vi "Dot_Plot_Sub.vi"(8 "Scaler plotted":string, 11 "Data":dbl[][](array[numeric])=[[-106.4208, 283.2907, 10.0, -0.027074, 202.4772, -73.9844, 9.9544], [-106.4108, 183.2989, 10.0, -0.06373, 202.4772, -73.9844, 9.9544], [-106.4104, 233.2978, 10.0, -0.10129, 202.4772, -73.9844, 9.9544], [-106.408, 333.302, 10.0, -0.09306, 202.4772, -73.9844, 9.9544], [138.8906, 606.731, 10.0, -0.003285, 202.4772, -73.9844, 9.9544], [238.889, 47.6577, 10.0, 0.004673, 202.4772, -73.9844, 9.9544], [238.8902, 606.729, 10.0, -0.003458, 202.4772, -73.9844, 9.9544], [288.8878, 47.6581, 10.0, 0.007221, 202.4772, -73.9844, 9.9544], [338.888, 606.73, 10.0, 0.004362, 202.4772, -73.9844, 9.9544], [338.891, 47.6626, 10.0, 0.006298, 202.4772, -73.9844, 9.9544], [388.892, -63.3583, 10.0, 4.5324, 202.4772, -73.9844, 9.9544], [388.892, 47.6606, 10.0, -0.008191, 202.4772, -73.9844, 9.9544], [438.889, 606.729, 10.0, -0.0028755, 202.4772, -73.9844, 9.9544], [438.89, -63.3577, 10.0, 4.2681, 202.4772, -73.9844, 9.9544], [438.891, 47.6608, 10.0, 0.026059, 202.4772, -73.9844, 9.9544], [488.89, 47.6614, 10.0, 0.14972, 202.4772, -73.9844, 9.9544], [488.892, -63.3599, 10.0, 6.2235, 202.4772, -73.9844, 9.9544], [538.89, -63.3596, 10.0, 7.0971, 202.4772, -73.9844, 9.9544], [538.891, 47.6597, 10.0, 0.7831, 202.4772, -73.9844, 9.9544], [538.893, 606.731, 10.0, 0.004097, 202.4772, -73.9844, 9.9544], [588.889, -63.3589, 10.0, 9.8267, 202.4772, -73.9844, 9.9544], [588.89, 47.659, 10.0, 1.4958, 202.4772, -73.9844, 9.9544], [638.889, 47.6597, 10.0, 2.7164, 202.4772, -73.9844, 9.9544], [638.89, 606.731, 10.0, 0.0016489, 202.4772, -73.9844, 9.9544], [638.891, -63.361, 10.0, 9.6904, 202.4772, -73.9844, 9.9544], [688.89, -63.3603, 10.0, 10.7752, 202.4772, -73.9844, 9.9544], [688.89, 47.6576, 10.0, 4.0933, 202.4772, -73.9844, 9.9544], [738.888, -63.3603, 10.0, 9.798, 202.4772, -73.9844, 9.9544], [738.889, 47.6583, 10.0, 5.4641, 202.4772, -73.9844, 9.9544], [738.89, 606.73, 10.0, 0.03667, 202.4772, -73.9844, 9.9544], [788.888, 47.659, 10.0, 6.5562, 202.4772, -73.9844, 9.9544], [788.889, -63.3624, 10.0, 9.7284, 202.4772, -73.9844, 9.9544], [838.888, -63.3617, 10.0, 9.2828, 202.4772, -73.9844, 9.9544], [838.888, 606.731, 10.0, 0.10792, 202.4772, -73.9844, 9.9544], [838.889, 47.6562, 10.0, 6.9452, 202.4772, -73.9844, 9.9544], [888.892, 47.6611, 10.0, 6.813, 202.4772, -73.9844, 9.9544], [888.892, -63.3575, 10.0, 8.8351, 202.4772, -73.9844, 9.9544], [938.888, 606.729, 10.0, 0.5974, 202.4772, -73.9844, 9.9544], [938.891, 47.6618, 10.0, 5.8719, 202.4772, -73.9844, 9.9544], [938.892, -63.3596, 10.0, 8.3492, 202.4772, -73.9844, 9.9544], [988.889, 47.6618, 10.0, 4.8748, 202.4772, -73.9844, 9.9544], [988.891, -63.3589, 10.0, 7.5502, 202.4772, -73.9844, 9.9544], [1038.888, 297.6587, 10.0, 3.1165, 202.4772, -73.9844, 9.9544], [1038.888, 97.6613, 10.0, 4.0692, 202.4772, -73.9844, 9.9544], [1038.888, 222.6594, 10.0, 2.9843, 202.4772, -73.9844, 9.9544], [1038.889, 147.6602, 10.0, 3.7073, 202.4772, -73.9844, 9.9544], [1038.889, 272.6583, 10.0, 3.0147, 202.4772, -73.9844, 9.9544], [1038.89, 72.6609, 10.0, 4.1188, 202.4772, -73.9844, 9.9544], [1038.89, 122.659, 10.0, 3.9763, 202.4772, -73.9844, 9.9544], [1038.89, 197.659, 10.0, 3.099, 202.4772, -73.9844, 9.9544], [1038.89, 247.6571, 10.0, 2.9194, 202.4772, -73.9844, 9.9544], [1038.89, 322.657, 10.0, 2.9534, 202.4772, -73.9844, 9.9544], [1038.89, 572.66, 10.0, 1.2565, 202.4772, -73.9844, 9.9544], [1038.89, 172.6578, 10.0, 3.3414, 202.4772, -73.9844, 9.9544], [1038.89, 447.662, 10.0, 2.4811, 202.4772, -73.9844, 9.9544], [1038.89, 522.662, 10.0, 1.3205, 202.4772, -73.9844, 9.9544], [1038.89, 47.6597, 10.0, 4.5287, 202.4772, -73.9844, 9.9544], [1038.89, -63.3589, 10.0, 6.8815, 202.4772, -73.9844, 9.9544], [1038.891, 372.662, 10.0, 2.8557, 202.4772, -73.9844, 9.9544], [1038.891, 497.66, 10.0, 1.5334, 202.4772, -73.9844, 9.9544], [1038.891, 547.66, 10.0, 1.2132, 202.4772, -73.9844, 9.9544], [1038.892, 422.661, 10.0, 2.7183, 202.4772, -73.9844, 9.9544], [1038.892, 472.661, 10.0, 1.9636, 202.4772, -73.9844, 9.9544], [1038.893, -7.8602, 10.0, 4.95, 202.4772, -73.9844, 9.9544], [1038.893, 347.662, 10.0, 2.9008, 202.4772, -73.9844, 9.9544], [1038.893, 606.731, 10.0, 1.1868, 202.4772, -73.9844, 9.9544], [1038.893, 397.661, 10.0, 2.8316, 202.4772, -73.9844, 9.9544], [1138.89, 606.732, 10.0, 1.4995, 202.4772, -73.9844, 9.9544], [1238.891, 606.73, 10.0, 1.7166, 202.4772, -73.9844, 9.9544], [1338.89, 606.729, 10.0, 1.8307, 202.4772, -73.9844, 9.9544], [1438.888, 606.729, 10.0, 1.8125, 202.4772, -73.9844, 9.9544]]) -> ()   [LabVIEW 2015]
uses:
  <vilib>/Utility/miscctls.llb/LV3DPointTypeDef.ctl
  <vilib>/Utility/miscctls.llb/LVRGBAColorTypeDef.ctl
  Globals/Constants_global.vi
  <vilib>/picture/3D Picture Control/Helpers/Set Light (no reference).vi
  <vilib>/picture/3D Picture Control/Object/Add Object (reference).vi
  <vilib>/picture/3D Picture Control/Object/Create Object (drawable).vi
  Gen Trav/Route mapping/Route_mapping_global.vi
  <vilib>/picture/3D Picture Control/NI_3D Picture Control.lvlib
panel:
  in  "Font, Size & Style":T1={"Desired Font (Application)"=enum."User-specified Font", "[User-specified Font]"={"Font Name"="Arial", "Size"=18, "Strikeout?"=FALSE, "Italic?"=FALSE, "Underline?"=FALSE, "Outline?"=FALSE, "Shadow?"=FALSE, "Bold?"=FALSE, "Rotation Angle"=0.0}, "Horizontal Alignment"=1, "Vertical Alignment"=0} {"Vertical Alignment" items=["Bottom", "Top", "Baseline"]; "Horizontal Alignment" items=["Left", "Center", "Right"]; "[User-specified Font]"."Rotation Angle" format="%.2f"}
  in  "Text position":u16(ring) items=["Top", "Bottom"]
  in  "Path to save picture":path=path "C:/Users/Paul Nathan/Desktop/test.jpg"
  in  "Save Picture":bool
  in  "Lift Measurement Position":dbl
  in  "Camera Position":T2={"X"=-0.0, "Y"=0.001, "Z"=3000.0}
  in  "Auto Camera Position":bool=TRUE
  in  "Bar Plot":bool
  in  "Max column Height":i32=1000
  in  "Manual Range":bool
  in  "Dem Min":dbl
  in  "Dem Max":dbl
  out "min value":dbl=-0.10129
  out "max value":dbl=10.7752
  in  "stop":bool
  in  "Space File Opacity":dbl(slide)=0.5051546391752577 scale=0.0..1.0
  in  "STL Model Opacity":dbl(slide)=1.0 scale=0.0..1.0
  in  "Fixed Colour":u32(colorbox)=16860
  in  "Cube Size":sgl=20.0
  in  "Model rotation":sgl(knob) scale=-360.0..360.0
  in  "Camera Height":dbl(slide)=3000.0 scale=1000.0..5000.0
  in  "Y shift":dbl(slide) scale=-3000.0..3000.0
  in  "X shift":sgl(slide) scale=-3000.0..3000.0
  in  "Model rotation axis":cluster{"X":sgl, "Y":sgl, "Z":sgl}={"X"=0.0, "Y"=0.0, "Z"=1.0}
  in  "Lock to plan view":bool=TRUE
  in  "Up Direction":T2={"X"=0.0, "Y"=0.0, "Z"=1.0}
  in  "Target":T2={"X"=-0.0, "Y"=-0.0, "Z"=0.0}
  in  "Browse CAD Model":path=path "C:/EnFlo Software/Anemometry/Anemometry Sub Vis/Templates/Diplos2.stl"
  in  "STL Model Colour":u32(colorbox)=16448250
  in  "Measurement\n Color Ramp":u32[](array[colorbox])=[16711680, 16776960, 6618880, 0]
  in  "Radius":sgl=20.0
  in  "Space File Color":u32(colorbox)=9868950
  out "3D Picture Control":refnum<vi>(3d-picture)
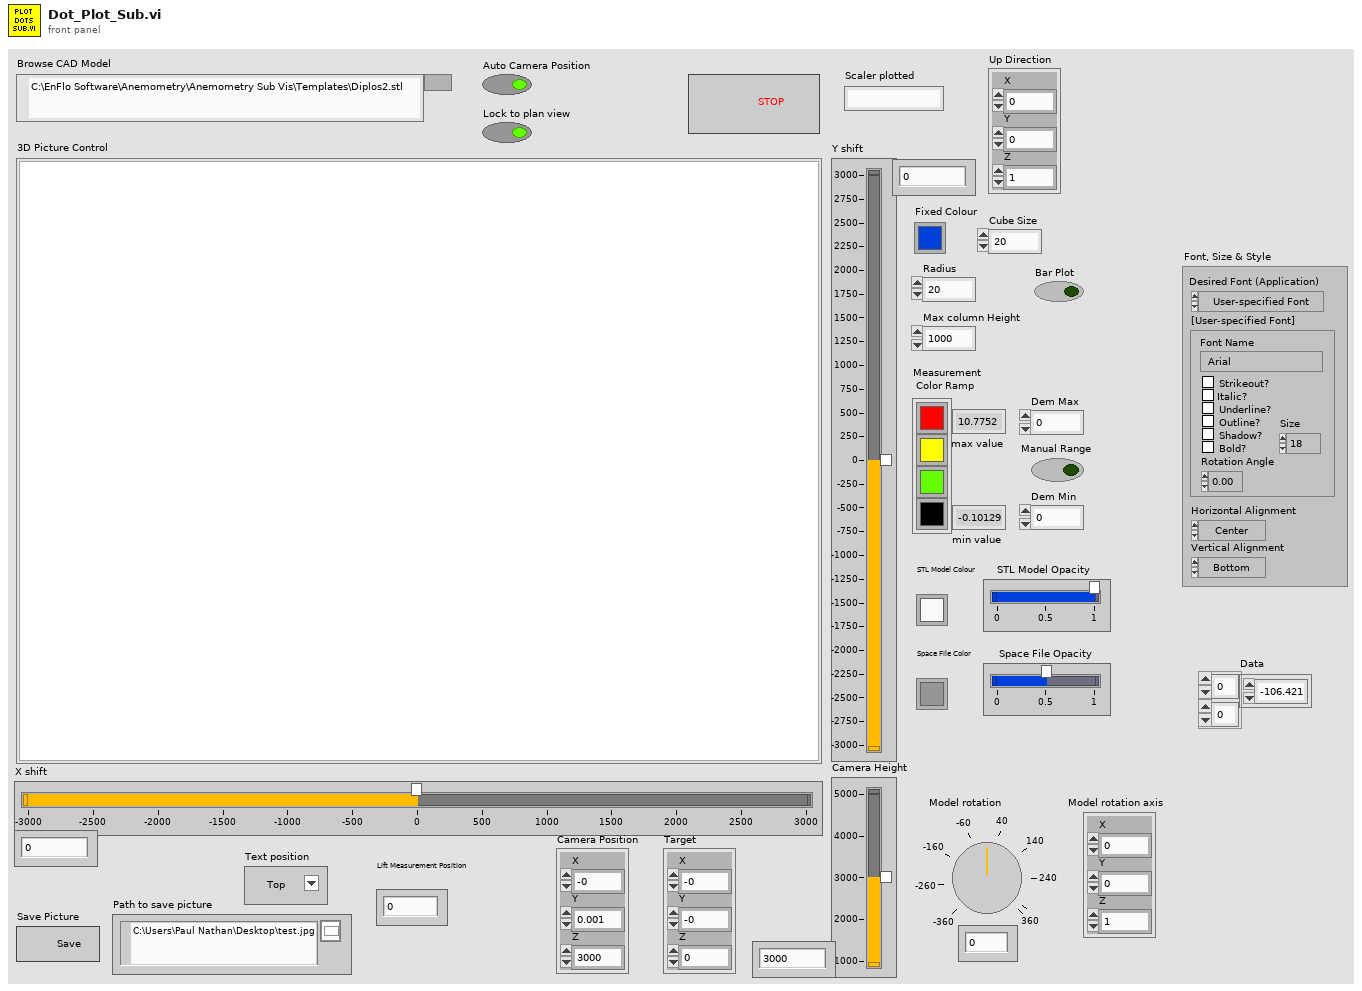
[diagram p1: front panel]
types:
  T1 = cluster{"Desired Font (Application)":enum16{"User-specified Font", "Application Font", "System Font", "Dialog Font"}, "[User-specified Font]":cluster{"Font Name":string, "Size":i16, "Strikeout?":bool, "Italic?":bool, "Underline?":bool, "Outline?":bool, "Shadow?":bool, "Bold?":bool, "Rotation Angle":dbl}, "Horizontal Alignment":i16, "Vertical Alignment":i16}
  T2 = typedef "LV3DPointTypeDef.ctl" = cluster{"X":sgl, "Y":sgl, "Z":sgl}
  T3 = enum16{"Inherit Value", "Points", "Wireframe", "Polygons"}
  T4 = enum16{"Inherit Value", "No Culling", "Cull Back Face", "Cull Front Face", "Cull Both Faces"}
  T5 = enum16{"Inherit Value", "Counterclockwise", "Clockwise"}
  T6 = typedef "LVRGBAColorTypeDef.ctl" = cluster{"Red":sgl, "Green":sgl, "Blue":sgl, "Alpha":sgl}
  T7 = typedef "Triangle.ctl" = cluster{"V0":sgl[], "V1":sgl[], "V2":sgl[], "E0":sgl[], "E1":sgl[], "E2":sgl[], "n^":sgl[], "nE0^":sgl[], "nE1^":sgl[], "nE2^":sgl[]}
  T8 = typedef "Exclude_cluster.ctl" = cluster{"Sizes":T9, "Name":string, "Exclude Type":T10}
  T9 = typedef "Box_size.ctl" = cluster{"Max":sgl, "Min":sgl}[]
  T10 = typedef "Exclusion_type.ctl" = enum16{"Exclude completely", "Allow only vertical moves"}
  T11 = typedef "imagedata.ctl" = cluster{"image type":i32, "image depth":i32, "image":u8[], "mask":u8[], "colors":u32[], "Rectangle":cluster{"left":i16, "top":i16, "right":i16, "bottom":i16}}
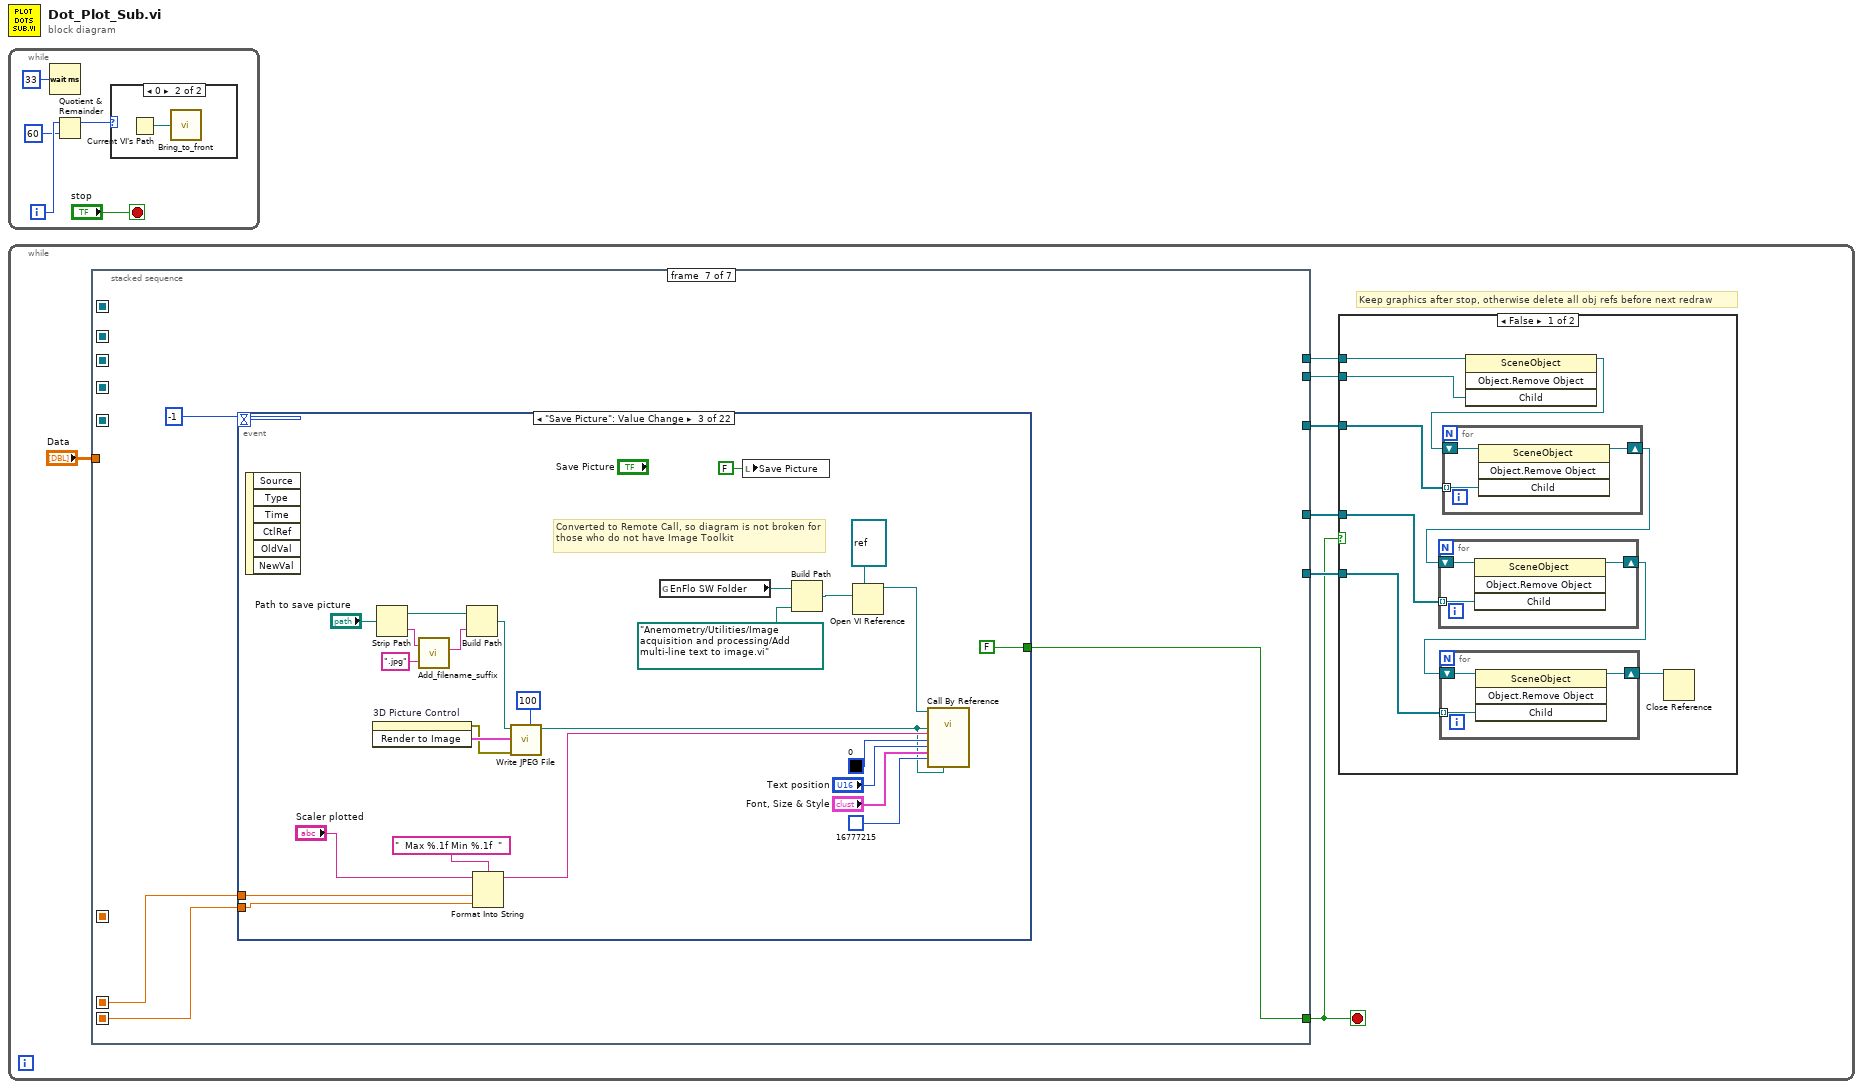
[diagram p0: block diagram]
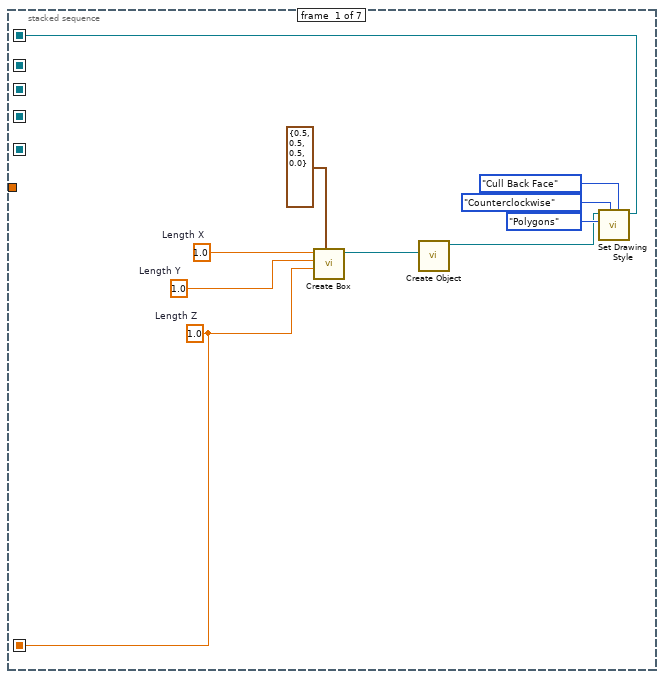
[diagram p4: hidden frame]
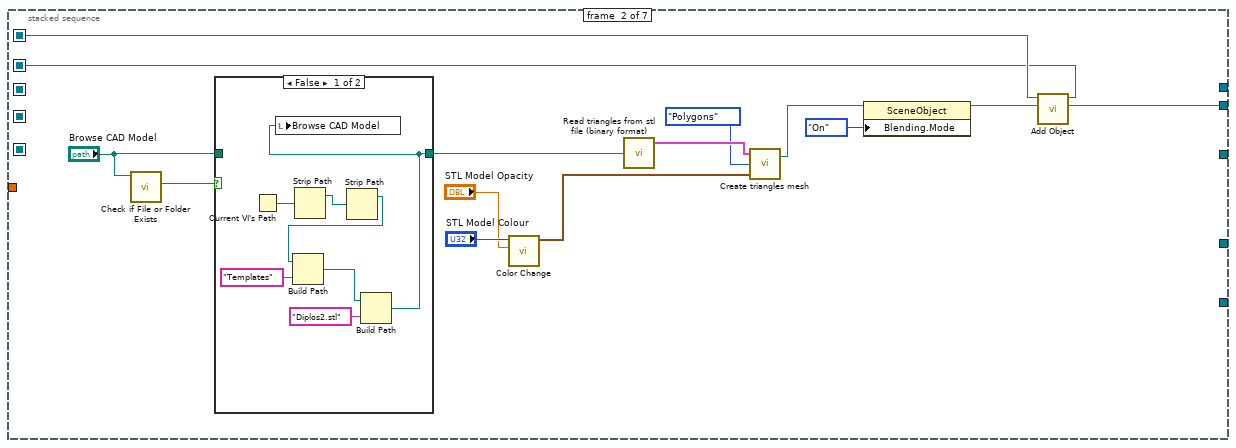
[diagram p5: hidden frame]
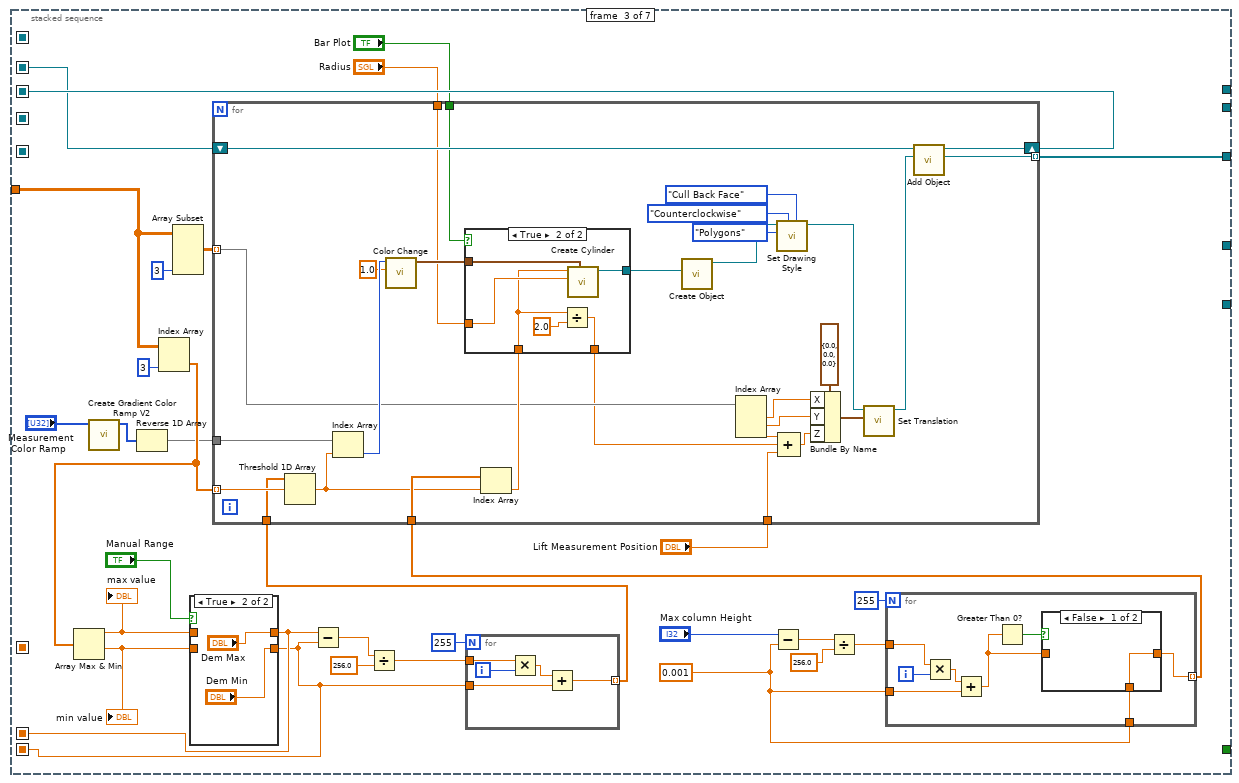
[diagram p7: hidden frame]
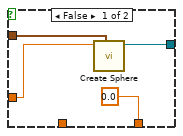
[diagram p10: hidden frame]
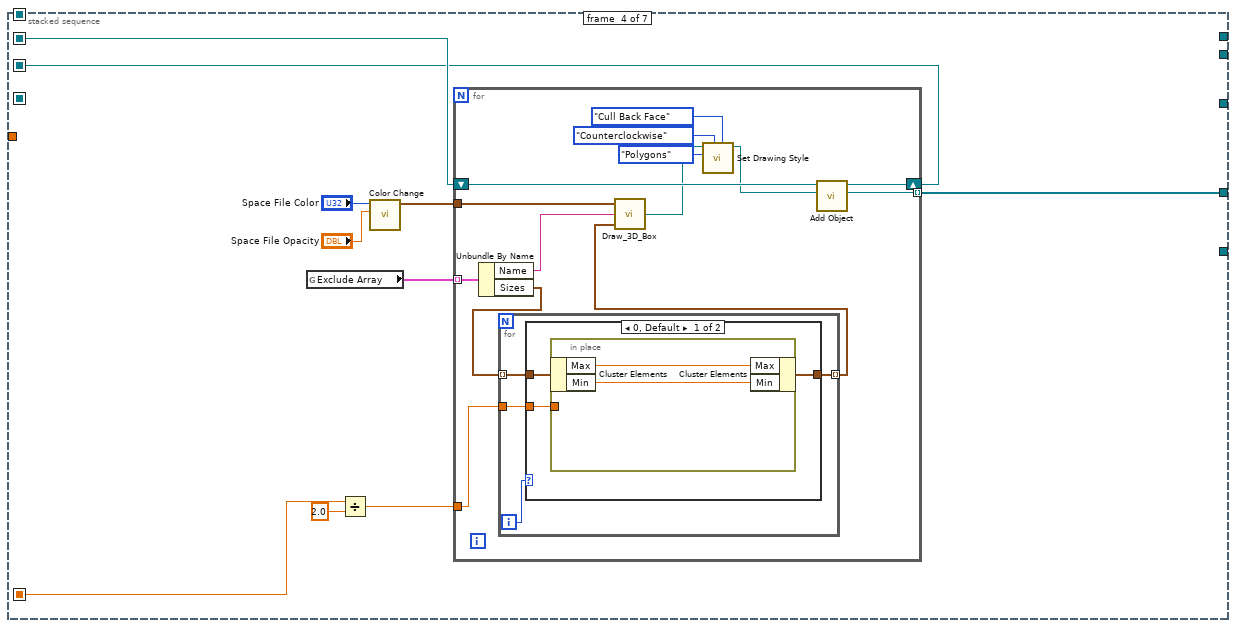
[diagram p11: hidden frame]
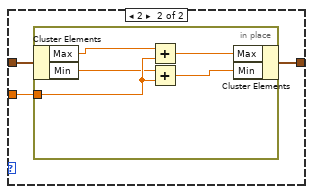
[diagram p12: hidden frame]
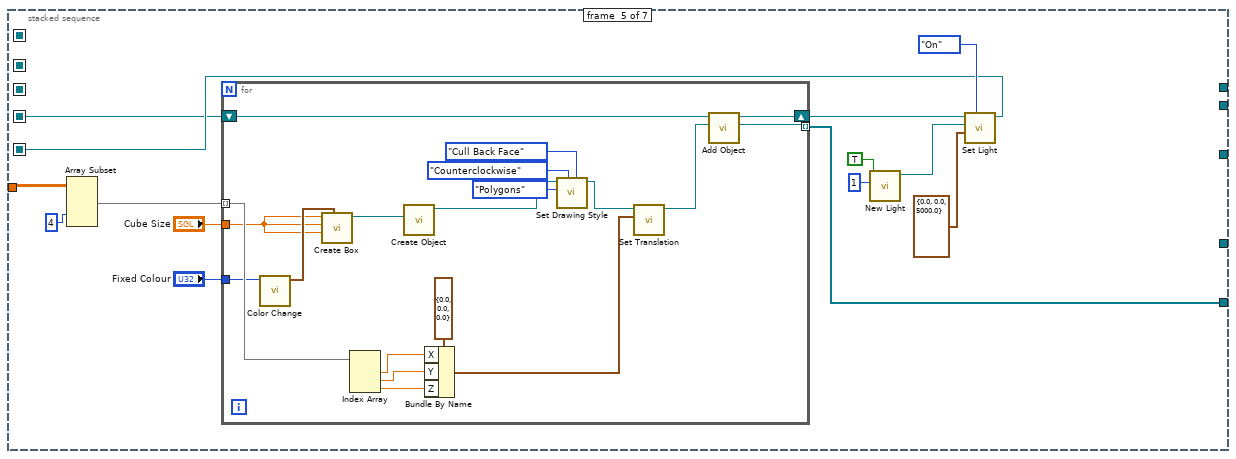
[diagram p13: hidden frame]
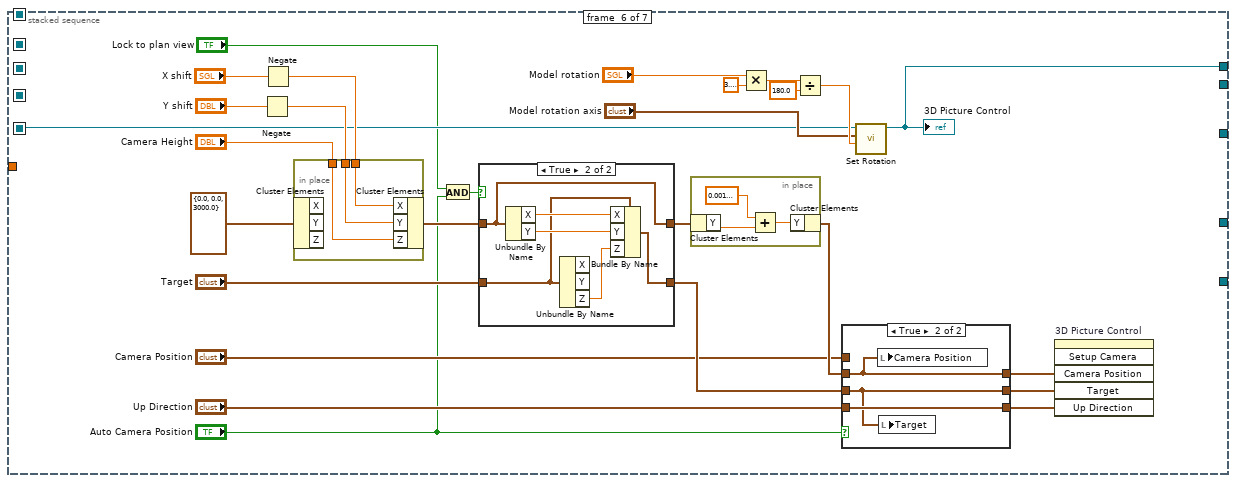
[diagram p14: hidden frame]
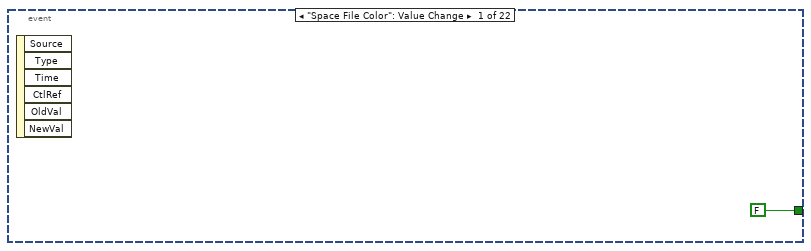
[diagram p17: hidden frame]
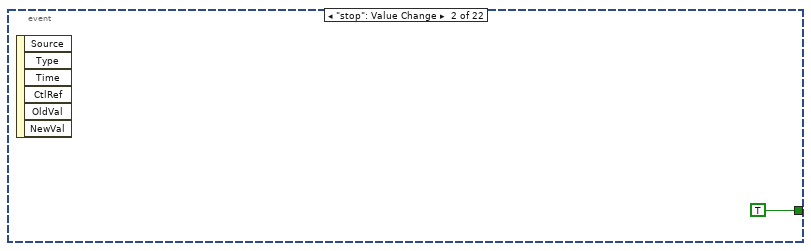
[diagram p18: hidden frame]
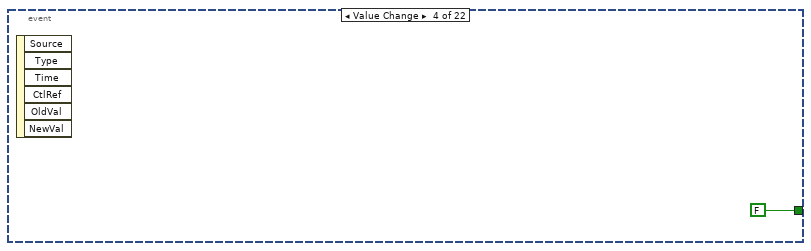
[diagram p19: hidden frame]
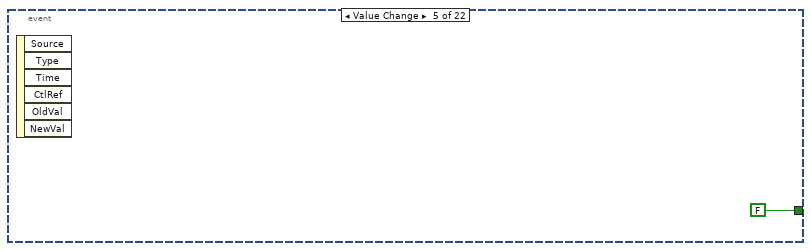
[diagram p20: hidden frame]
diagram:
  n1 = while {
    i -> [w3]
    stop <- "stop" stop-if-true
    n2 = Wait (ms)(milliseconds to wait=u32 33) -> ()  [unwired: 1 out]
    n3 = Quotient & Remainder(x=w3, y=60) -> (x-y*floor(x/y)=w1:i32)  [unwired: 1 out]
    n4 = case shown="0" w1 {
      frame Default {
      }
      frame 0 {
        n5 = Current VI's Path() -> (path=w6:path)
        n6 = call "Bring_to_front.vi"("path"=w6) -> ()
      }
    }
  }
  n7 = while {
    stop <- w7 stop-if-true
    # "Keep graphics after stop, otherwise delete all obj refs before next redraw"
    n8 = stacked-sequence {
      seq-local: [w32 _ _ _ _ _ _] -> [_ w55 _ _ _ _ _]
      seq-local: [w41 _ _ _ _ _ _] -> [_ _ _ w157 _ _ _]
      seq-local: [_ w54 _ _ _ _ _] -> [_ _ w81 _ _ _ _]
      seq-local: [_ _ w82 _ _ _ _] -> [_ _ _ w159 _ _ _]
      seq-local: [_ _ _ _ w199 _ _] -> [_ _ _ _ _ w237 _]
      seq-local: [_ _ _ w158 _ _ _] -> [_ _ _ _ w198 _ _]
      seq-local: [_ _ w65 _ _ _ _] -> [_ _ _ _ _ _ w276]
      seq-local: [_ _ w64 _ _ _ _] -> [_ _ _ _ _ _ w275]
      tunnel: "Data" -> [_ _ w85 _ w202 _ _]
      tunnel: [_ _ _ _ _ _ w278] -> w7
      tunnel: [_ w42 _ _ _ _ _] -> w11
      tunnel: [_ _ w69 _ _ _ _] -> w12
      tunnel: [_ _ _ w154 _ _ _] -> w9
      tunnel: [_ _ _ _ w197 _ _] -> w8
      tunnel: [_ _ _ _ _ w235 _] -> w10
      frame #0 {
        w41 = sgl 1.0  # Length Z
        w38 = sgl 1.0  # Length Y
        w39 = sgl 1.0  # Length X
        n9 = call <vilib>:"Create Box.vi"("Color"=T6 {"Red"=0.5, "Green"=0.5, "Blue"=0.5, "Alpha"=0.0} ("Color 2"), "Length Z"=w41, "Length Y"=w38, "Length X"=w39) -> ("New Box Refnum"=w37:refnum<vi>)  [unwired: 6 in, 1 out]
        n10 = call-poly <vilib>:"Create Object.vi"("Geometry"=w37) -> ("Scene:New Object"=w33:refnum<vi>)  [unwired: 9 in, 1 out]
        n11 = call <vilib>:"Set Drawing Style.vi"("Face Culling Mode"=T4."Cull Back Face", "Frontface Mode"=T5."Counterclockwise", "Mode"=T3."Polygons", "Scene Object In"=w33) -> ("Scene Object Out"=w32:refnum<vi>)  [unwired: 6 in, 1 out]
      }
      frame #1 {
        n12 = call <vilib>:"Check if File or Folder Exists.vi"("path"="Browse CAD Model") -> ("file or folder exists?"=w52:bool)  [unwired: 8 in, 2 out]
        n13 = case shown="False" w52 {
          tunnel: [w56 w63] -> w48
          tunnel: "Browse CAD Model" -> [_ w63]
          frame False {
            n14 = Current VI's Path() -> (path=w62:path)
            n15 = Strip Path(path=w62) -> (stripped path=w61:path)  [unwired: 1 out]
            n16 = Strip Path(path=w61) -> (stripped path=w60:path)  [unwired: 1 out]
            n17 = Build Path(base path=w60, name or relative path="Templates") -> (appended path=w58:path)
            n18 = Build Path(base path=w58, name or relative path="Diplos2.stl") -> (appended path=w56:path)
            n19 = local write "Browse CAD Model"(w56) -> ()
          }
          frame True {
          }
        }
        n20 = call <vilib>:"Color Change.vi"("Alpha"="STL Model Opacity", "Color"="STL Model Colour") -> ("RGBA"=w45:cluster{"R":sgl, "G":sgl, "B":sgl, "A":sgl})  [unwired: 9 in]
        n21 = call "Read triangles from stl file (binary format).vi"("STL file path"=w48) -> ("Triangles array"=w47:T7[])  [unwired: 2 out]
        n22 = call "Create triangles mesh.vi"("Colour"=w45, "Render mode"=T3."Polygons", "Triangles array"=w47) -> ("Triangle mesh out"=w43:refnum<vi>)  [unwired: 1 out]
        n23 = property class="SceneObject"(reference=w43, "Blending.Mode"=enum16{"Inherit Value", "Off", "On"}."On" ("Blending:Mode")) -> (reference out=w49:refnum<vi>)  [unwired: 1 in, 1 out]
        n24 = call-poly <vilib>:"Add Object.vi"("New Object In"=w49, "Scene Object In"=w55) -> ("New Object Out"=w42:refnum<vi>, "Scene Object Out"=w54:refnum<vi>)  [unwired: 7 in, 1 out]
      }
      frame #2 {
        w72 = 0.001
        n25 = call "Create Gradient Color Ramp V2.vi"("Color Array"="Measurement\n Color Ramp") -> ("Color Table"=w93:u32[])  [unwired: 8 in, 2 out]
        n26 = Reverse 1D Array(array=w93) -> (reversed array=w90:u32[])
        n27 = Index Array(array=w85, index (col)=3 ("disabled index (col)")) -> (element=w91:dbl[])  [unwired: 1 in]
        n28 = Array Max & Min(array=w91) -> (max value=w79:dbl, min value=w78:dbl)  [unwired: 2 out]
        "max value" <- w79
        "min value" <- w78
        n29 = Array Subset(array=w85, length (col)=3 ("length")) -> (w83:dbl[][])  [unwired: 3 in]
        n30 = case shown="True" "Manual Range" {
          tunnel: [w106 "Dem Max"] -> w65
          tunnel: w79 -> [w106 _]
          tunnel: [w105 "Dem Min"] -> w64
          tunnel: w78 -> [w105 _]
          frame False {
          }
          frame True {
          }
        }
        n31 = Subtract(x=w65, y=w64) -> (x-y=w89:dbl)
        n32 = Divide(x=w89, y=256.0) -> (x/y=w87:dbl)
        n33 = for {
          N: 255 -> [_]
          tunnel: w87 -> [w112]
          tunnel: w64 -> [w110]
          tunnel: [w109] -> w71 mode=indexing
          i -> [w113]
          n34 = Multiply(x=w112, y=w113) -> (x*y=w111:dbl)
          n35 = Add(x=w111, y=w110) -> (x+y=w109:dbl)
        }
        n36 = Subtract(x="Max column Height", y=w72) -> (x-y=w74:dbl)
        n37 = Divide(x=w74, y=256.0) -> (x/y=w76:dbl)
        n38 = for {
          N: 255 -> [_]
          tunnel: w76 -> [w101]
          tunnel: w72 -> [w99]
          tunnel: [w98] -> w73 mode=indexing
          tunnel: w72 -> [w95]
          i -> [w102]
          n39 = Multiply(x=w101, y=w102) -> (x*y=w100:dbl)
          n40 = Add(x=w100, y=w99) -> (x+y=w97:dbl)
          n41 = Greater Than 0?(x=w97) -> (x > 0?=w96:bool)
          n42 = case shown="False" w96 {
            tunnel: [w103 w104] -> w98
            tunnel: w97 -> [_ w104]
            tunnel: w95 -> [w103 _]
            frame False {
            }
            frame True {
            }
          }
        }
        n43 = for {
          shift-right: [w138] -> w82
          shift-left: w81 -> [w139]
          tunnel: w73 -> [w133]
          tunnel: w91 -> [w131] mode=indexing
          tunnel: w90 -> [w132]
          tunnel: w83 -> [w129] mode=indexing
          tunnel: w71 -> [w130]
          tunnel: [w123] -> w69 mode=indexing
          tunnel: "Bar Plot" -> [w116]
          tunnel: "Radius" -> [w115]
          tunnel: "Lift Measurement Position" -> [w114]
          n44 = Threshold 1D Array(2:w131, 3:w130) -> (0:w128:dbl)  [unwired: 1 in]
          n45 = Index Array(array=w132, index=w128) -> (element=w135:u32)
          n46 = call <vilib>:"Color Change.vi"("Alpha"=1.0, "Color"=w135) -> ("RGBA"=w136:cluster{"R":sgl, "G":sgl, "B":sgl, "A":sgl})  [unwired: 9 in]
          n47 = Index Array(array=w133, index=w128) -> (element=w134:dbl)
          n48 = case shown="True" w116 {
            tunnel: w136 -> [w146 w153]
            tunnel: [w145 w152] -> w124
            tunnel: w115 -> [w147 w151]
            tunnel: w134 -> [_ w148]
            tunnel: [0.0 w149] -> w125
            frame False {
              n49 = call <vilib>:"Create Sphere.vi"("Color"=w146, "Radius"=w147) -> ("New Sphere Refnum"=w145:refnum<vi>)  [unwired: 8 in, 1 out]
            }
            frame True {
              n50 = Divide(x=w148, y=2.0) -> (x/y=w149:dbl)
              n51 = call <vilib>:"Create Cylinder.vi"("Color"=w153, "Radius"=w151, "Height"=w148) -> ("New Cylinder Refnum"=w152:refnum<vi>)  [unwired: 7 in, 1 out]
            }
          }
          n52 = call-poly <vilib>:"Create Object.vi"("Geometry"=w124) -> ("Scene:New Object"=w121:refnum<vi>)  [unwired: 9 in, 1 out]
          n53 = Index Array(array=w129) -> (element #1=w142:dbl, element #2=w143:dbl, element #3=w127:dbl)  [unwired: 3 in]
          n54 = call <vilib>:"Set Drawing Style.vi"("Face Culling Mode"=T4."Cull Back Face", "Frontface Mode"=T5."Counterclockwise", "Mode"=T3."Polygons", "Scene Object In"=w121) -> ("Scene Object Out"=w120:refnum<vi>)  [unwired: 6 in, 1 out]
          n55 = Compound Arithmetic op=ADD(w127, w125, w114) -> (w126:dbl)
          n56 = Bundle By Name(cluster=cluster{"X":sgl, "Y":sgl, "Z":sgl} {"X"=0.0, "Y"=0.0, "Z"=0.0} ("Translation"), "X"=w142, "Y"=w143, "Z"=w126) -> (w140:cluster{"X":sgl, "Y":sgl, "Z":sgl})
          n57 = call <vilib>:"Set Translation.vi"("Translation"=w140, "Scene Object"=w120) -> ("Translated Object"=w137:refnum<vi>)  [unwired: 8 in, 1 out]
          n58 = call-poly <vilib>:"Add Object.vi"("New Object In"=w137, "Scene Object In"=w139) -> ("New Object Out"=w123:refnum<vi>, "Scene Object Out"=w138:refnum<vi>)  [unwired: 7 in, 1 out]
        }
      }
      frame #3 {
        n59 = global read "Route_mapping_global.vi" "Exclude Array"() -> (w163:T8[])
        n60 = Divide(x=w157, y=sgl 2.0) -> (x/y=w160:sgl)
        n61 = call <vilib>:"Color Change.vi"("Alpha"="Space File Opacity", "Color"="Space File Color") -> ("RGBA"=w155:cluster{"R":sgl, "G":sgl, "B":sgl, "A":sgl})  [unwired: 9 in]
        n62 = for {
          tunnel: w163 -> [w177] mode=indexing
          tunnel: w155 -> [w176]
          tunnel: w160 -> [w174]
          shift-right: [w170] -> w158
          shift-left: w159 -> [w171]
          tunnel: [w169] -> w154 mode=indexing
          n63 = Unbundle By Name(w177) -> ("Name"=w175:string, "Sizes"=w173:T9)
          n64 = for {
            tunnel: w174 -> [w181]
            tunnel: w173 -> [w180] mode=indexing
            tunnel: [w179] -> w172 mode=indexing
            i -> [w178]
            n65 = case shown="0, Default" w178 {
              tunnel: w181 -> [w184 w189]
              tunnel: w180 -> [w183 w188]
              tunnel: [w182 w187] -> w179
              frame 0, Default {
                n66 = in-place {
                  in-place-border: w184 -> [_]
                  n67 = in-place-cluster #1(w183) -> ("Max"=w186:sgl, "Min"=w185:sgl)
                  n68 = in-place-cluster #1("Max"=w186, "Min"=w185) -> (w182:cluster{"Max":sgl, "Min":sgl})
                }
              }
              frame 2 {
                n69 = in-place {
                  in-place-border: w189 -> [w194]
                  n70 = in-place-cluster #2(w188) -> ("Max"=w191:sgl, "Min"=w190:sgl)
                  n71 = Add(x=w191, y=w194) -> (x+y=w193:sgl)
                  n72 = Add(x=w190, y=w194) -> (x+y=w192:sgl)
                  n73 = in-place-cluster #2("Max"=w193, "Min"=w192) -> (w187:cluster{"Max":sgl, "Min":sgl})
                }
              }
            }
          }
          n74 = call "Draw_3D_Box.vi"("Box Coordinates"=w172, "Name"=w175, "Color"=w176) -> ("Translated Object"=w165:refnum<vi>)
          n75 = call <vilib>:"Set Drawing Style.vi"("Face Culling Mode"=T4."Cull Back Face", "Frontface Mode"=T5."Counterclockwise", "Mode"=T3."Polygons", "Scene Object In"=w165) -> ("Scene Object Out"=w164:refnum<vi>)  [unwired: 6 in, 1 out]
          n76 = call-poly <vilib>:"Add Object.vi"("New Object In"=w164, "Scene Object In"=w171) -> ("New Object Out"=w169:refnum<vi>, "Scene Object Out"=w170:refnum<vi>)  [unwired: 7 in, 1 out]
        }
      }
      frame #4 {
        n77 = Array Subset(array=w202, index (col)=4 ("length")) -> (w201:dbl[][])  [unwired: 3 in]
        n78 = for {
          tunnel: w201 -> [w218] mode=indexing
          shift-right: [w221] -> w203
          shift-left: w198 -> [w222]
          tunnel: [w216] -> w197 mode=indexing
          tunnel: "Fixed Colour" -> [w210]
          tunnel: "Cube Size" -> [w209]
          n79 = call <vilib>:"Color Change.vi"("Color"=w210) -> ("RGBA"=w219:cluster{"R":sgl, "G":sgl, "B":sgl, "A":sgl})  [unwired: 10 in]
          n80 = call <vilib>:"Create Box.vi"("Color"=w219, "Length Z"=w209, "Length Y"=w209, "Length X"=w209) -> ("New Box Refnum"=w217:refnum<vi>)  [unwired: 6 in, 1 out]
          n81 = Index Array(array=w218) -> (element #1=w225:dbl, element #2=w226:dbl, element #3=w227:dbl)  [unwired: 3 in]
          n82 = call-poly <vilib>:"Create Object.vi"("Geometry"=w217) -> ("Scene:New Object"=w212:refnum<vi>)  [unwired: 9 in, 1 out]
          n83 = Bundle By Name(cluster=cluster{"X":sgl, "Y":sgl, "Z":sgl} {"X"=0.0, "Y"=0.0, "Z"=0.0} ("Translation"), "X"=w225, "Y"=w226, "Z"=w227) -> (w223:cluster{"X":sgl, "Y":sgl, "Z":sgl})
          n84 = call <vilib>:"Set Drawing Style.vi"("Face Culling Mode"=T4."Cull Back Face", "Frontface Mode"=T5."Counterclockwise", "Mode"=T3."Polygons", "Scene Object In"=w212) -> ("Scene Object Out"=w211:refnum<vi>)  [unwired: 6 in, 1 out]
          n85 = call <vilib>:"Set Translation.vi"("Translation"=w223, "Scene Object"=w211) -> ("Translated Object"=w220:refnum<vi>)  [unwired: 8 in, 1 out]
          n86 = call-poly <vilib>:"Add Object.vi"("New Object In"=w220, "Scene Object In"=w222) -> ("New Object Out"=w216:refnum<vi>, "Scene Object Out"=w221:refnum<vi>)  [unwired: 7 in, 1 out]
        }
        n87 = call <vilib>:"New Light.vi"("Light Number"=1, "At Infinity"=TRUE) -> ("New Light Refnum"=w205:refnum<vi>)  [unwired: 8 in, 1 out]
        n88 = call-poly <vilib>:"Set Light.vi"("Light State"=enum16{"Inherit Value", "Off", "On"}."On", "Position"=T2 {"X"=0.0, "Y"=0.0, "Z"=5000.0}, "Light Refnum In"=w205, "Scene Object In"=w203) -> ("Scene Object Out"=w199:refnum<vi>)  [unwired: 6 in, 1 out]
      }
      frame #5 {
        n89 = Negate(x="Y shift") -> (-x=w240:dbl)
        n90 = Negate(x="X shift") -> (-x=w241:sgl)
        n91 = in-place {
          in-place-border: w241 -> [w263]
          in-place-border: w240 -> [w262]
          in-place-border: "Camera Height" -> [w261]
          n92 = in-place-cluster #3(T2 {"X"=0.0, "Y"=0.0, "Z"=3000.0} ("Camera Position")) -> ()  [unwired: 3 out]
          n93 = in-place-cluster #3("X"=w263, "Y"=w262, "Z"=w261) -> (w244:T2)
        }
        n94 = And(x="Lock to plan view", y="Auto Camera Position") -> (x .and. y?=w229:bool)
        n95 = case shown="True" w229 {
          tunnel: w244 -> [w267 w269]
          tunnel: "Target" -> [w268 w272]
          tunnel: [w268 w270] -> w252
          tunnel: [w267 w269] -> w251
          frame False {
          }
          frame True {
            n96 = Unbundle By Name(w269) -> ("X"=w274:sgl, "Y"=w273:sgl)
            n97 = Unbundle By Name(w272) -> ("Z"=w271:sgl)  [unwired: 2 out]
            n98 = Bundle By Name(cluster=w272, "X"=w274, "Y"=w273, "Z"=w271) -> (w270:T2)
          }
        }
        n99 = in-place {
          n100 = in-place-cluster #4(w251) -> ("Y"=w266:sgl)
          n101 = Add(x=sgl 0.001, y=w266) -> (x+y=w265:sgl)
          n102 = in-place-cluster #4("Y"=w265) -> (w250:T2)
        }
        n103 = Multiply(x="Model rotation", y=sgl 3.1415927) -> (x*y=w249:sgl)
        n104 = Divide(x=w249, y=sgl 180.0) -> (x/y=w246:sgl)
        n105 = case shown="True" "Auto Camera Position" {
          tunnel: "Up Direction" -> [w257 w260]
          tunnel: w252 -> [w256 w258]
          tunnel: w250 -> [_ w259]
          tunnel: [w255 w259] -> w234
          tunnel: [w256 w258] -> w233
          tunnel: [w257 w260] -> w232
          tunnel: "Camera Position" -> [w255 _]
          frame False {
          }
          frame True {
            n106 = local write "Camera Position"(w259) -> ()
            n107 = local write "Target"(w258) -> ()
          }
        }
        n108 = call <vilib>:"Set Rotation.vi"("Angle"=w246, "Axis"="Model rotation axis", "Scene Object"=w237) -> ("Rotated Scene Object"=w235:refnum<vi>)  [unwired: 7 in, 1 out]
        "3D Picture Control" <- w235
        n109 = invoke on="3D Picture Control" class="SceneGraphDisp (strict)" method="Setup Camera"("Camera Position"=w234, "Target"=w233, "Up Direction"=w232) -> ()  [unwired: 3 in, 6 out]
      }
      frame #6 {
        n110 = event shown="[2] \"Save Picture\": Value Change" {
          selector: _ -> [_ _ _ _ _ _ _ _ _ _ _ _ _ _ _ _ _ _ _ _ _ _]
          dyn-events: _ -> [_ _ _ _ _ _ _ _ _ _ _ _ _ _ _ _ _ _ _ _ _ _]
          timeout: -1 -> [_ _ _ _ _ _ _ _ _ _ _ _ _ _ _ _ _ _ _ _ _ _]
          tunnel: [FALSE ("stop") TRUE ("stop") FALSE ("stop") FALSE ("stop") FALSE ("stop") FALSE ("stop") FALSE ("stop") FALSE ("stop") FALSE ("stop") FALSE ("stop") FALSE ("stop") FALSE ("stop") FALSE ("stop") FALSE ("stop") FALSE ("stop") FALSE ("stop") FALSE ("stop") FALSE ("stop") FALSE ("stop") FALSE ("stop") FALSE ("stop") FALSE ("stop")] -> w278
          tunnel: w276 -> [_ _ w295 _ _ _ _ _ _ _ _ _ _ _ _ _ _ _ _ _ _ _]
          tunnel: w275 -> [_ _ w281 _ _ _ _ _ _ _ _ _ _ _ _ _ _ _ _ _ _ _]
          event "Space File Color": Value Change {
            n111 = event-data() -> ()  [unwired: 1 in, 6 out]
          }
          event "stop": Value Change {
            n112 = event-data() -> ()  [unwired: 1 in, 6 out]
          }
          event "Save Picture": Value Change {
            # "Converted to Remote Call, so diagram is not broken for those who do not have Image Toolkit"
            n113 = event-data() -> ()  [unwired: 1 in, 6 out]
            n114 = invoke on="3D Picture Control" class="SceneGraphDisp (strict)" method="Render to Image"() -> (error out=w305:errorcluster, "Get Image"=w306:T11)  [unwired: 3 in, 1 out]
            n115 = Strip Path(path="Path to save picture") -> (stripped path=w297:path, name=w299:string)
            n116 = call "Add_filename_suffix.vi"("Filename"=w299, "Suffix to add"=".jpg") -> ("Filename out"=w298:string)  [unwired: 3 out]
            n117 = Build Path(base path=w297, name or relative path=w298) -> (appended path=w296:path)
            n118 = Format Into String(format string="  Max %.1f Min %.1f  ", initial string="Scaler plotted", w295, w281) -> (resulting string=w284:string)  [unwired: 1 in, 1 out]
            n119 = call <vilib>:"Write JPEG File.vi"("quality (80)"=100, "error in (no error)"=w305, "image data"=w306, "path to JPEG file"=w296) -> ("path"=w283:path)  [unwired: 6 in, 1 out]
            n120 = global read "Constants_global.vi" "EnFlo SW Folder"() -> (w290:path)
            n121 = local write "Save Picture"(FALSE ("Save Picture")) -> ()
            n122 = Build Path(base path=w290, name or relative path=path "Anemometry/Utilities/Image acquisition and processing/Add multi-line text to image.vi") -> (appended path=w293:path)
            n123 = Open VI Reference(type specifier VI Refnum (for type only)=refnum<vi> refnum, vi path=w293) -> (vi reference=w292:refnum<vi>)  [unwired: 2 in, 3 out]
            n124 = call-by-ref "?"(reference=w292, "Text to add"=w284, "Image load path"=w283, "Text colour"=u32 0, "Text position"="Text position", "Font, Size & Style"="Font, Size & Style", "Background colour"=u32 16777215, "Image save path"=w283) -> ()  [unwired: 9 in, 3 out]
          }
          event Value Change {
            n125 = event-data() -> ()  [unwired: 1 in, 6 out]
          }
          event Value Change {
            n126 = event-data() -> ()  [unwired: 1 in, 6 out]
          }
          event Timeout {
            n127 = event-data() -> ()  [unwired: 1 in, 3 out]
          }
          event "Radius": Value Change {
            n128 = event-data() -> ()  [unwired: 1 in, 6 out]
          }
          event "Measurement\n Color Ramp": Value Change {
            n129 = event-data() -> ()  [unwired: 1 in, 6 out]
          }
          event "STL Model Colour": Value Change {
            n130 = event-data() -> ()  [unwired: 1 in, 6 out]
          }
          event "Lock to plan view": Value Change {
            n131 = event-data() -> ()  [unwired: 1 in, 6 out]
          }
          event "X shift": Value Change {
            n132 = event-data() -> ()  [unwired: 1 in, 6 out]
          }
          event "Y shift": Value Change {
            n133 = event-data() -> ()  [unwired: 1 in, 6 out]
          }
          event "Camera Height": Value Change {
            n134 = event-data() -> ()  [unwired: 1 in, 6 out]
          }
          event "Bar Plot": Value Change {
            n135 = event-data() -> ()  [unwired: 1 in, 6 out]
          }
          event "Auto Camera Position": Value Change {
            n136 = event-data() -> ()  [unwired: 1 in, 6 out]
          }
          event "Model rotation": Value Change {
            n137 = event-data() -> ()  [unwired: 1 in, 6 out]
          }
          event "STL Model Opacity": Value Change {
            n138 = event-data() -> ()  [unwired: 1 in, 6 out]
          }
          event "Space File Opacity": Value Change {
            n139 = event-data() -> ()  [unwired: 1 in, 6 out]
          }
          event "Dem Max": Value Change {
            n140 = event-data() -> ()  [unwired: 1 in, 6 out]
          }
          event "Dem Min": Value Change {
            n141 = event-data() -> ()  [unwired: 1 in, 6 out]
          }
          event "Manual Range": Value Change {
            n142 = event-data() -> ()  [unwired: 1 in, 6 out]
          }
          event "Cube Size": Value Change {
            n143 = event-data() -> ()  [unwired: 1 in, 6 out]
          }
        }
      }
    }
    n144 = case shown="False" w7 {
      tunnel: w12 -> [w22 _]
      tunnel: w11 -> [w21 _]
      tunnel: w10 -> [w20 _]
      tunnel: w9 -> [w18 _]
      tunnel: w8 -> [w16 _]
      frame False {
        n145 = invoke class="SceneObject" method="Object.Remove Object"(reference=w20, "Child"=w21) -> (reference out=w19:refnum<vi>)  [unwired: 2 in, 3 out]
        n146 = for {
          tunnel: w22 -> [w31] mode=indexing
          shift-right: [w29] -> w17
          shift-left: w19 -> [w30]
          n147 = invoke class="SceneObject" method="Object.Remove Object"(reference=w30, "Child"=w31) -> (reference out=w29:refnum<vi>)  [unwired: 2 in, 3 out]
        }
        n148 = for {
          tunnel: w18 -> [w28] mode=indexing
          shift-right: [w26] -> w15
          shift-left: w17 -> [w27]
          n149 = invoke class="SceneObject" method="Object.Remove Object"(reference=w27, "Child"=w28) -> (reference out=w26:refnum<vi>)  [unwired: 2 in, 3 out]
        }
        n150 = for {
          tunnel: w16 -> [w25] mode=indexing
          shift-right: [w23] -> w14
          shift-left: w15 -> [w24]
          n151 = invoke class="SceneObject" method="Object.Remove Object"(reference=w24, "Child"=w25) -> (reference out=w23:refnum<vi>)  [unwired: 2 in, 3 out]
        }
        n152 = Close Reference(reference=w14) -> ()  [unwired: 1 in, 1 out]
      }
      frame True {
      }
    }
  }
